vi "ParseHistory.vi"(1 "History Data":cluster{"ori_X":dbl, "ori_Y":dbl, "ori_Z":dbl}[](array[cluster])) -> (0 "Array":dbl[][](array[numeric]))   [LabVIEW 2014]
doc: "Returns a 2D array containing the history of the waveform given. The expected input is an array of cluster elements.\n\nEach of these elements contains 3 double (numeric) values. At first a 2D array of 50 rows, or less if the history length (=HL) is smaller and 3 columns for each one of the cluster's components. The last 2 samples from the history are discarded since an auto-stop might add noise. Then, for each 0<i<50(or less) element of the history[HL-50(or less)-2+i] unbundle the doubles and store them in the i-th row of the 2D array"
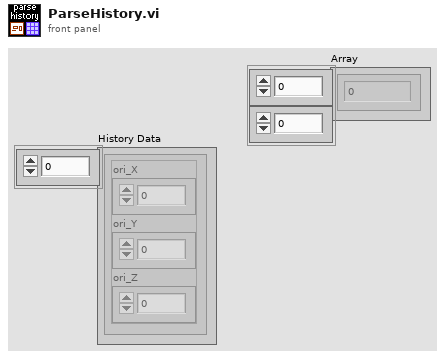
[diagram p1: front panel]
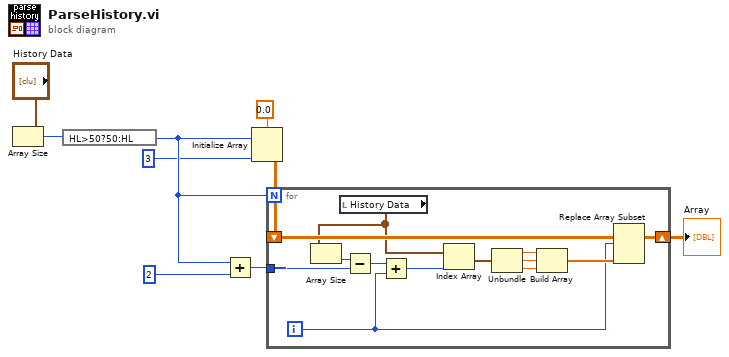
[diagram p0: block diagram]
diagram:
  n1 = Array Size(array="History Data") -> (size(s)=w5:i32)
  n2 = expression code="HL>50?50:HL"(w5) -> (w8:i32)
  n3 = Add(x=w8, y=2) -> (x+y=w7:i32)
  n4 = Initialize Array(0.0 ("element"), w8, 3 ("dimension size")) -> (w2:dbl[][])
  n5 = for {
    N: w8 -> [_]
    shift-right: [w16] -> w9
    shift-left: w2 -> [w17]
    tunnel: w7 -> [w14]
    i -> [w11]
    n6 = local read "History Data"() -> (w10:cluster{"ori_X":dbl, "ori_Y":dbl, "ori_Z":dbl}[])
    n7 = Array Size(array=w10) -> (size(s)=w15:i32)
    n8 = Subtract(x=w15, y=w14) -> (x-y=w13:i32)
    n9 = Add(x=w13, y=w11) -> (x+y=w12:i32)
    n10 = Index Array(array=w10, index=w12) -> (element=w22:cluster{"ori_X":dbl, "ori_Y":dbl, "ori_Z":dbl})
    n11 = Unbundle(w22) -> ("ori_X"=w21:dbl, "ori_Y"=w20:dbl, "ori_Z"=w19:dbl)
    n12 = Build Array(w21, w20, w19) -> (w18:dbl[])
    n13 = Replace Array Subset(array=w17, new element=w18, index (row)=w11) -> (w16:dbl[][])  [unwired: 1 in]
  }
  "Array" <- w9
